vi "ImportScan.vi"(0 "Experiment in":refnum<class "Experiment.lvclass">, 9 "scan_idx":dbl, 11 "error in (no error)":errorcluster, 12 "Ball Motion":bool=TRUE, 13 "Video":bool=TRUE, 14 "Analog Signals":bool=TRUE) -> (4 "Experiment out":refnum<class "Experiment.lvclass">, 15 "error out":errorcluster)   [LabVIEW 2014, in "Experiment.lvclass"]
uses:
  Experiment.lvclass
  Experiment.lvclass/Experiment.ctl
  Database/Database.lvclass
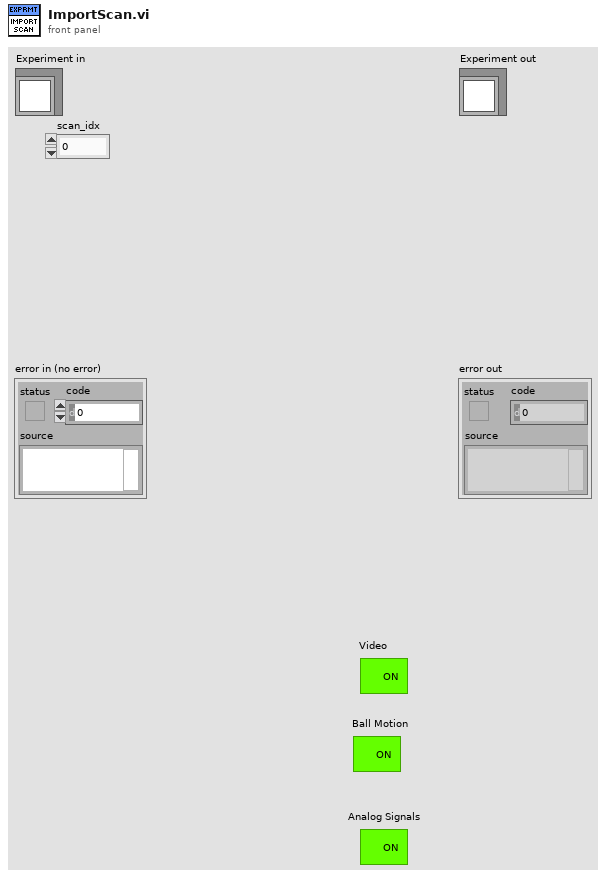
[diagram p1: front panel]
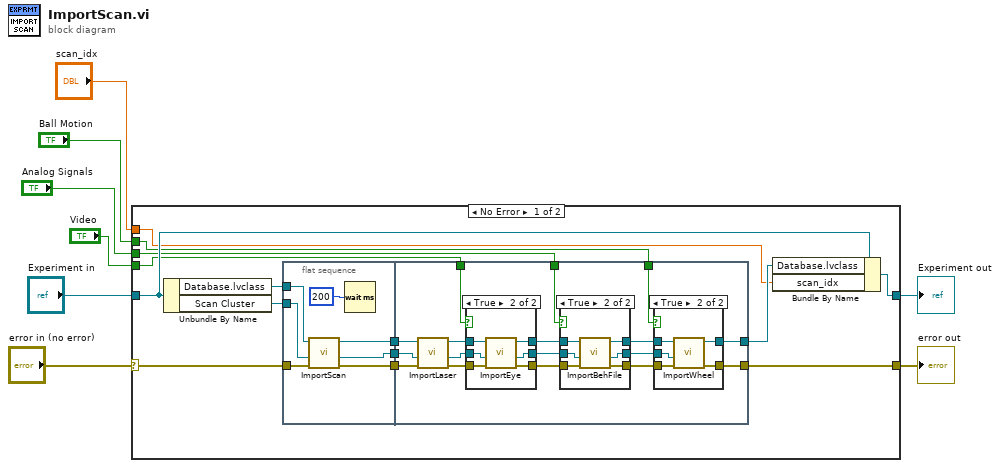
[diagram p0: block diagram]
diagram:
  n1 = case shown="No Error" "error in (no error)" {
    selector: "error in (no error)" -> [w9 w73]
    tunnel: [w16 w73] -> w7
    tunnel: [w20 w72] -> w5
    tunnel: "Experiment in" -> [w21 w72]
    tunnel: "scan_idx" -> [w14 _]
    tunnel: "Analog Signals" -> [w11 _]
    tunnel: "Ball Motion" -> [w12 _]
    tunnel: "Video" -> [w13 _]
    frame No Error {
      n2 = Unbundle By Name(w21) -> ("Database.lvclass"=w18:refnum<class "Database.lvclass">, "Scan Cluster"=w10:refnum<vi>)
      n3 = flat-sequence {
        tunnel: [w29] -> w19
        tunnel: w18 -> [w28]
        tunnel: w9 -> [w27]
        tunnel: [w26] -> w17
        tunnel: [w25] -> w15
        tunnel: w10 -> [w24]
        tunnel: [w43] -> w22
        tunnel: w19 -> [w46]
        tunnel: w17 -> [w42]
        tunnel: [w38] -> w16
        tunnel: w15 -> [w34]
        tunnel: w13 -> [w32]
        tunnel: w12 -> [w31]
        tunnel: w11 -> [w30]
        frame #0 {
          n4 = call-dynamic "ImportScan.vi"("error in (no error)"=w27, "reference"=w24, "Database in"=w28) -> ("error out"=w26:errorcluster, "reference 2"=w25:refnum<vi>, "Database out"=w29:refnum<class "Database.lvclass">)  [unwired: 6 in]
          n5 = Wait (ms)(milliseconds to wait=u32 200) -> ()  [unwired: 1 out]
        }
        frame #1 {
          n6 = call-dynamic "ImportLaser.vi"("error in (no error)"=w42, "reference"=w34, "Database in"=w46) -> ("error out"=w41:errorcluster, "reference 2"=w35:refnum<vi>, "Database out"=w45:refnum<class "Database.lvclass">)  [unwired: 6 in]
          n7 = case shown="True" w32 {
            tunnel: w45 -> [w65 w71]
            tunnel: w41 -> [w64 w69]
            tunnel: [w64 w68] -> w40
            tunnel: [w63 w67] -> w36
            tunnel: w35 -> [w63 w66]
            tunnel: [w65 w70] -> w33
            frame False {
            }
            frame True {
              n8 = call-dynamic "ImportEye.vi"("error in (no error)"=w69, "reference"=w66, "Database in"=w71) -> ("error out"=w68:errorcluster, "reference 2"=w67:refnum<vi>, "Database out"=w70:refnum<class "Database.lvclass">)  [unwired: 6 in]
            }
          }
          n9 = case shown="True" w30 {
            tunnel: w33 -> [w56 w62]
            tunnel: [w56 w61] -> w44
            tunnel: w40 -> [w55 w60]
            tunnel: [w55 w59] -> w39
            tunnel: [w54 w58] -> w37
            tunnel: w36 -> [w54 w57]
            frame False {
            }
            frame True {
              n10 = call-dynamic "ImportBehFile.vi"("error in (no error)"=w60, "reference"=w57, "Database in"=w62) -> ("error out"=w59:errorcluster, "reference 2"=w58:refnum<vi>, "Database out"=w61:refnum<class "Database.lvclass">)  [unwired: 6 in]
            }
          }
          n11 = case shown="True" w31 {
            tunnel: w44 -> [w48 w53]
            tunnel: [w48 w52] -> w43
            tunnel: w39 -> [w47 w51]
            tunnel: [w47 w50] -> w38
            tunnel: w37 -> [_ w49]
            frame False {
            }
            frame True {
              n12 = call-dynamic "ImportWheel.vi"("error in (no error)"=w51, "reference"=w49, "Database in"=w53) -> ("error out"=w50:errorcluster, "Database out"=w52:refnum<class "Database.lvclass">)  [unwired: 6 in, 1 out]
            }
          }
        }
      }
      n13 = Bundle By Name(cluster=w21, "Database.lvclass"=w22, "scan_idx"=w14) -> (w20:refnum<class "Experiment.lvclass">)
    }
    frame Error {
    }
  }
  "error out" <- w7
  "Experiment out" <- w5
